vi "Plot Helper (Vector).vi"(8 "error in (no error)":errorcluster, 9 "z vector":sgl[](array[numeric]), 10 "y vector":sgl[](array[numeric])) -> (0 "error out":errorcluster, 3 "3D Plot lvclass Array out":refnum<class "3D Plot Datatype.lvclass">[](array[class]))   [LabVIEW 2020, in "3D Bar Datatype.lvclass"]
doc: "Generates a plot of vertical bars."
uses:
  <vilib>/Math Plots/3D Math Plots/3D Bar/3D Bar Datatype/3D Bar Datatype.lvclass
  <vilib>/Math Plots/3D Math Plots/3D Plot/3D Plot Datatype/3D Plot Datatype.lvclass
  e:/builds/penguin/labview/branches/2020/dev/dist/vi.lib/Math Plots/3D Math Plots/3D Plot/3D Plot Datatype/3D Plot Datatype.lvclass
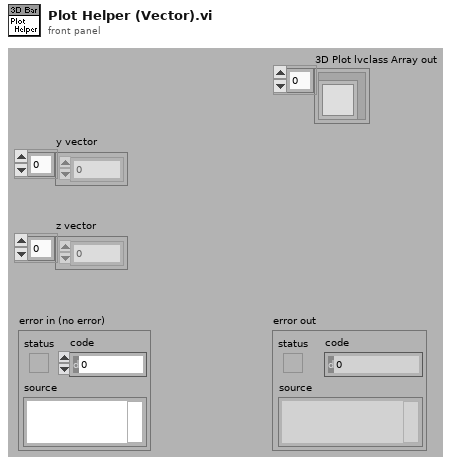
[diagram p1: front panel]
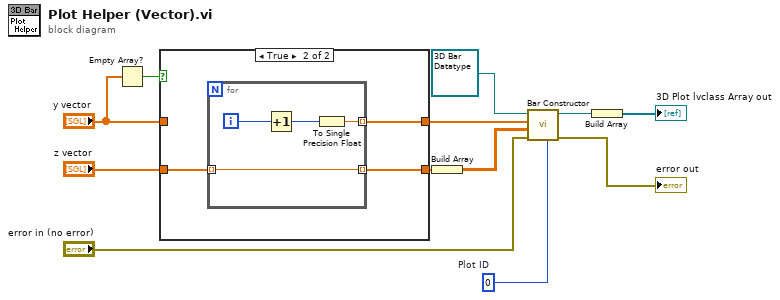
[diagram p0: block diagram]
diagram:
  w3 = 0  # Plot ID
  n1 = Empty Array?(array="y vector") -> (empty?=w8:bool)
  n2 = case shown="True" w8 {
    tunnel: "y vector" -> [w16 _]
    tunnel: "z vector" -> [w13 w21]
    tunnel: [w15 w19] -> w7
    tunnel: [w14 w20] -> w5
    frame False {
      # "All 2 vectors should have the same dimension.\nThat dimension should be the smallest one."
      n3 = for {
        tunnel: [w18] -> w14 mode=indexing
        tunnel: w13 -> [w18] mode=indexing
        tunnel: w16 -> [w17] mode=indexing
        tunnel: [w17] -> w15 mode=indexing
      }
    }
    frame True {
      n4 = for {
        tunnel: [w25] -> w20 mode=indexing
        tunnel: w21 -> [w25] mode=indexing
        tunnel: [w22] -> w19 mode=indexing
        i -> [w24]
        n5 = Increment(x=w24) -> (x+1=w23:i32)
        n6 = To Single Precision Float(number=w23) -> (single precision float=w22:sgl)
      }
    }
  }
  n7 = Build Array(w5) -> (w4:sgl[][])
  n8 = call-dynamic "Bar Constructor.vi"("Plot ID"=w3, "error in (no error)"="error in (no error)", "z matrix"=w4, "y vector"=w7, "3D Bar Datatype.lvclass in"=refnum<class "3D Bar Datatype.lvclass"> refnum ("3D Mesh Datatype.lvclass")) -> ("error out"=→"error out":errorcluster, "3D Bar Datatype.lvclass out"=w2:refnum<class "3D Bar Datatype.lvclass">)  [unwired: 1 in, 4 out]
  n9 = Build Array(w2) -> (→"3D Plot lvclass Array out":refnum<class "3D Bar Datatype.lvclass">[])
